vi "RSZVB Get Coupled Markers.vi"(8 "error in (no error)":errorcluster {"code" format="%.0x"}, 9 "Marker (1)":i32=1, 10 "Channel (Trace) (1)":i32=1, 11 "VISA session":refnum<visa-resource-name>) -> (0 "error out":errorcluster {"code" format="%.0x"}, 2 "Marker Coupled":bool, 3 "dup VISA session":refnum<visa-resource-name>)   [LabVIEW 2011]
doc: "This VI returns if the markers of all traces in the active setup are coupled to the markers of trace no. <Ch/Tr>.\n\nRemote-control command(s):\nCALCulate<Ch/Tr>:MARKer<Mk>:COUPled[:STATe]?"
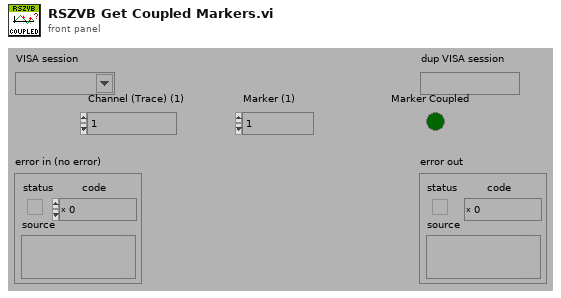
[diagram p1: front panel]
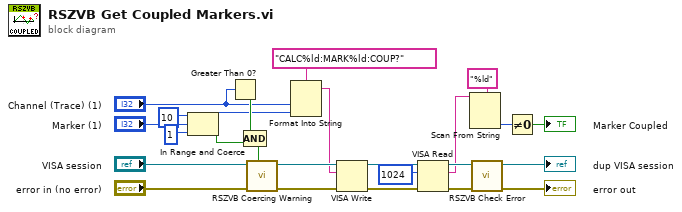
[diagram p0: block diagram]
diagram:
  n1 = In Range and Coerce(upper limit=10, x="Marker (1)", lower limit=1) -> (coerced(x)=w10:i32, In Range?=w11:bool)
  n2 = Greater Than 0?(x="Channel (Trace) (1)") -> (x > 0?=w14:bool)
  n3 = Compound Arithmetic op=AND(w14, w11) -> (w16:bool)
  n4 = call "RSZVB Coercing Warning.vi"("In Range?"=w16, "error in (no error)"="error in (no error)", "VISA session"="VISA session") -> ("error out"=w17:errorcluster, "dup VISA session"=w18:refnum<visa-resource-name>)  [unwired: 7 in]
  n5 = Format Into String(format string="CALC%ld:MARK%ld:COUP?", "Channel (Trace) (1)", w10) -> (resulting string=w15:string)  [unwired: 2 in, 1 out]
  n6 = VISA Write(VISA resource name=w18, write buffer=w15, error in (no error)=w17) -> (VISA resource name out=w8:refnum<visa-resource-name>, error out=w9:errorcluster)  [unwired: 1 out]
  n7 = VISA Read(VISA resource name=w8, byte count=u32 1024 ("byte count (0)"), error in (no error)=w9) -> (VISA resource name out=w24:refnum<visa-resource-name>, read buffer=w21:string, error out=w23:errorcluster)  [unwired: 1 out]
  n8 = Scan From String(format string="%ld", input string=w21) -> (output 1=w20:i32)  [unwired: 3 in, 3 out]
  n9 = call "RSZVB Check Error.vi"("error in (no error)"=w23, "VISA session"=w24) -> ("error out"=→"error out":errorcluster, "dup VISA session"=→"dup VISA session":refnum<visa-resource-name>)  [unwired: 8 in]
  n10 = Not Equal To 0?(x=w20) -> (x != 0?=→"Marker Coupled":bool)
